vi "Extrapolate Covariance.vi"(8 "Q":T1, 9 "F":T1, 11 "Covariance":T1) -> (3 "Predicted Covariance":T1)   [LabVIEW 2020]
uses:
  <vilib>/Analysis/Matrix/Datatypes/RealMatrix.ctl
  <vilib>/Analysis/7linalg.llb/Real Transpose Matrix.vi
  <vilib>/Analysis/baseanly.llb/Real A x B.vi
  <vilib>/Analysis/Matrix/Numeric/Add/Add - RM,RM.vi
  <vilib>/Analysis/NI_AALPro.lvlib
  <vilib>/Analysis/NI_AALBase.lvlib
  <vilib>/Analysis/Matrix/NI_Matrix.lvlib
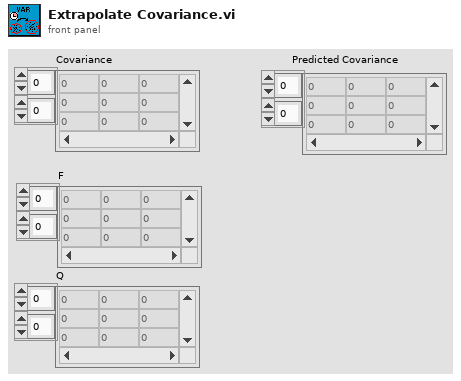
[diagram p1: front panel]
types:
  T1 = typedef "NI_Matrix.lvlib/RealMatrix.ctl" = dbl[][]
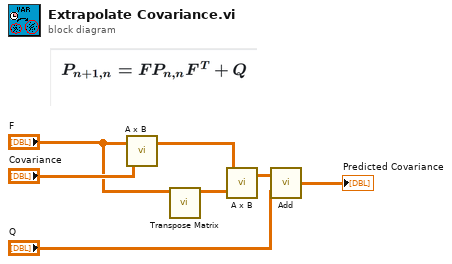
[diagram p0: block diagram]
diagram:
  n1 = call-poly <vilib>:"A x B.vi"("B"="Covariance", "A"="F") -> ("A x B"=w5:T1)  [unwired: 1 out]
  n2 = call-poly <vilib>:"Transpose Matrix.vi"("Input Matrix"="F") -> ("Matrix Transpose"=w4:T1)  [unwired: 9 in, 1 out]
  n3 = call-poly <vilib>:"A x B.vi"("B"=w4, "A"=w5) -> ("A x B"=w3:T1)  [unwired: 1 out]
  n4 = call-poly <vilib>:"Add.vi"("Real Matrix B"="Q", "Real Matrix A"=w3) -> ("A + B"=→"Predicted Covariance":T1)
